vi "Read Value.vi"(8 "error in (no error)":errorcluster, 11 "Boolean Parameter in":refnum<class "Boolean Parameter.lvclass">) -> (0 "error out":errorcluster, 2 "Value":bool, 3 "Boolean Parameter out":refnum<class "Boolean Parameter.lvclass">)   [LabVIEW 2019, in "CD Parameter Manager API.lvlib" / "Boolean Parameter.lvclass"]
uses:
  Boolean Parameter.lvclass
  Boolean Parameter.lvclass/Boolean Parameter.ctl
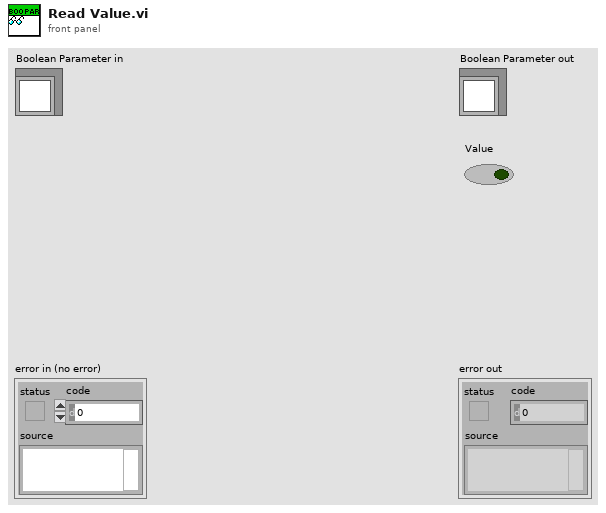
[diagram p1: front panel]
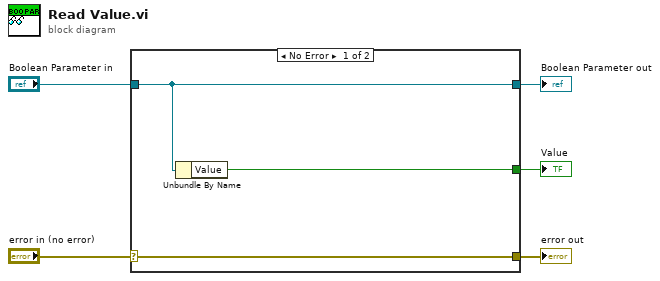
[diagram p0: block diagram]
diagram:
  n1 = case shown="No Error" "error in (no error)" {
    selector: "error in (no error)" -> [w8 w9]
    tunnel: [w8 w9] -> w4
    tunnel: [w7 w10] -> w2
    tunnel: "Boolean Parameter in" -> [w7 w10]
    tunnel: [w6 _] -> w1
    frame No Error {
      n2 = Unbundle By Name(w7) -> ("Value"=w6:bool)
    }
    frame Error {
    }
  }
  "error out" <- w4
  "Boolean Parameter out" <- w2
  "Value" <- w1
